vi "FTW-JSON-LexicalScan-IsDigit.vi"(0 "JSON String":T1, 11 "error in":errorcluster) -> (4 "JSON String Out":T1, 8 "Is Digit":bool, 15 "error out":errorcluster)   [LabVIEW 2015]
uses:
  FTW-JSON-LexicalScan.ctl
panel:
  # "Inputs"
  # "Outputs"
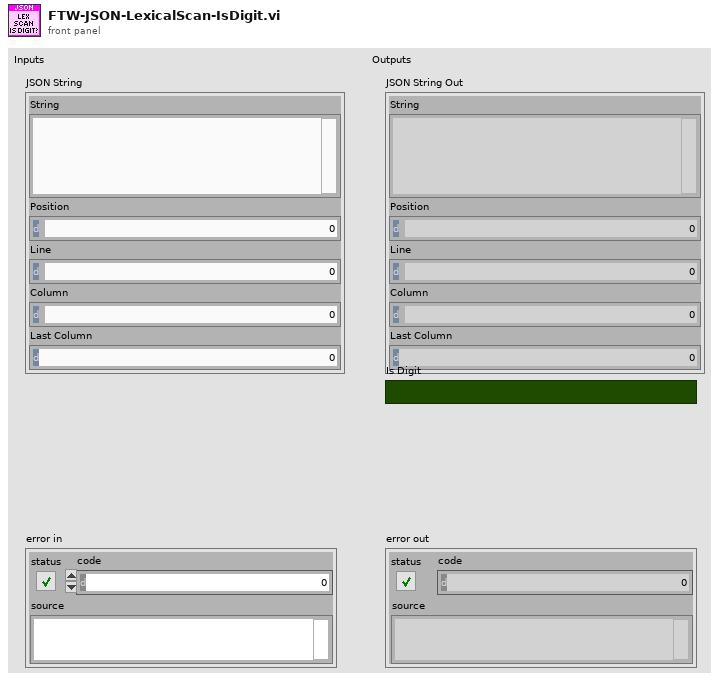
[diagram p1: front panel]
types:
  T1 = typedef "FTW-JSON-LexicalScan.ctl" = cluster{"String":string, "Position":i32, "Line":i32, "Column":i32, "Last Column":i32}
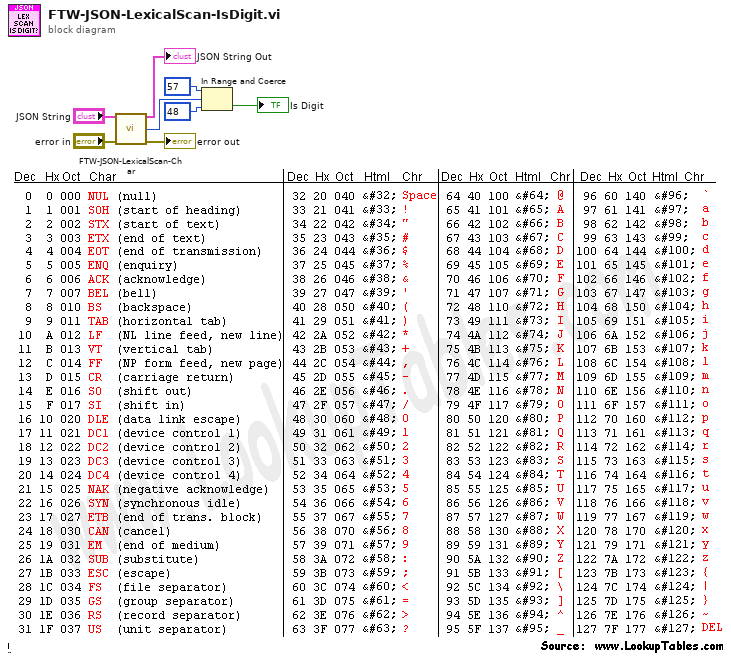
[diagram p0: block diagram]
diagram:
  n1 = call "FTW-JSON-LexicalScan-Char.vi"("JSON String"="JSON String", "error in"="error in") -> ("JSON String Out"=→"JSON String Out":T1, "Char"=w1:u8, "error out"=→"error out":errorcluster)  [unwired: 11 in]
  n2 = In Range and Coerce(upper limit=u8 57, x=w1, lower limit=u8 48) -> (In Range?=→"Is Digit":bool)  [unwired: 1 out]
